vi "HFRR ADV v07.vi"() -> ()   [LabVIEW 2025] (continued)
        n800 = local write "CAMERA ROI MIN TEMP"(TRUE ("CAMERA ROI MIN TEMP")) -> ()
      }
      frame "Compare Files" {
        n801 = local read "LIVE FEED MIN TEMP"() -> (w1178:bool)
        n802 = local write "LIVE FEED MAX TEMP"(TRUE ("LIVE FEED MAX TEMP")) -> ()
        n803 = local read "CAMERA ROI MIN TEMP"() -> (w1176:bool)
        n804 = case shown="True" w1178 {
          selector: w1178 -> [_ w1185]
          frame False {
          }
          frame True {
            n805 = Not(x=w1185) -> (.not. x?=w1184:bool)
            n806 = local write "LIVE FEED MIN TEMP"(w1184) -> ()
            n807 = call "CAMERA LIVE FEED FGV.vi"("Enum - Menu"=CAMERA_LIVE_FEED_ENUM."CAMERA MINIMIZE") -> ()  [unwired: 9 in, 2 out]
          }
        }
        n808 = case shown="True" w1176 {
          selector: w1176 -> [_ w1182]
          frame False {
          }
          frame True {
            n809 = Not(x=w1182) -> (.not. x?=w1181:bool)
            n810 = local write "CAMERA ROI MIN TEMP"(w1181) -> ()
            n811 = call "IMAGE ANALYSIS.vi"("Enum"=POST_ANALYSIS_ENUM."MINIMIZE UI") -> ()  [unwired: 9 in, 2 out]
          }
        }
        n812 = local write "CAMERA ROI MAX TEMP"(TRUE ("CAMERA ROI MAX TEMP")) -> ()
      }
      frame "About" {
        n813 = local read "LIVE FEED MIN TEMP"() -> (w1188:bool)
        n814 = local write "LIVE FEED MAX TEMP"(TRUE ("LIVE FEED MAX TEMP")) -> ()
        n815 = local read "CAMERA ROI MIN TEMP"() -> (w1187:bool)
        n816 = case shown="True" w1188 {
          selector: w1188 -> [_ w1195]
          frame False {
          }
          frame True {
            n817 = Not(x=w1195) -> (.not. x?=w1194:bool)
            n818 = local write "LIVE FEED MIN TEMP"(w1194) -> ()
            n819 = call "CAMERA LIVE FEED FGV.vi"("Enum - Menu"=CAMERA_LIVE_FEED_ENUM."CAMERA MINIMIZE") -> ()  [unwired: 9 in, 2 out]
          }
        }
        n820 = case shown="True" w1187 {
          selector: w1187 -> [_ w1192]
          frame False {
          }
          frame True {
            n821 = Not(x=w1192) -> (.not. x?=w1191:bool)
            n822 = local write "CAMERA ROI MIN TEMP"(w1191) -> ()
            n823 = call "IMAGE ANALYSIS.vi"("Enum"=POST_ANALYSIS_ENUM."MINIMIZE UI") -> ()  [unwired: 9 in, 2 out]
          }
        }
        n824 = local write "CAMERA ROI MAX TEMP"(TRUE ("CAMERA ROI MIN TEMP")) -> ()
      }
      frame "Advance" {
        n825 = local read "LIVE FEED MIN TEMP"() -> (w1198:bool)
        n826 = local write "LIVE FEED MAX TEMP"(TRUE ("LIVE FEED MAX TEMP")) -> ()
        n827 = local read "CAMERA ROI MIN TEMP"() -> (w1196:bool)
        n828 = case shown="True" w1198 {
          selector: w1198 -> [_ w1205]
          frame False {
          }
          frame True {
            n829 = Not(x=w1205) -> (.not. x?=w1204:bool)
            n830 = local write "LIVE FEED MIN TEMP"(w1204) -> ()
            n831 = call "CAMERA LIVE FEED FGV.vi"("Enum - Menu"=CAMERA_LIVE_FEED_ENUM."CAMERA MINIMIZE") -> ()  [unwired: 9 in, 2 out]
          }
        }
        n832 = local write "CAMERA ROI MAX TEMP"(TRUE ("CAMERA ROI MAX TEMP")) -> ()
        n833 = case shown="True" w1196 {
          selector: w1196 -> [_ w1202]
          frame False {
          }
          frame True {
            n834 = Not(x=w1202) -> (.not. x?=w1201:bool)
            n835 = local write "CAMERA ROI MIN TEMP"(w1201) -> ()
            n836 = call "IMAGE ANALYSIS.vi"("Enum"=POST_ANALYSIS_ENUM."MINIMIZE UI") -> ()  [unwired: 9 in, 2 out]
          }
        }
      }
      frame "Mooha" {
        n837 = local read "LIVE FEED MIN TEMP"() -> (w1208:bool)
        n838 = local write "LIVE FEED MAX TEMP"(TRUE ("LIVE FEED MAX TEMP")) -> ()
        n839 = local read "CAMERA ROI MIN TEMP"() -> (w1206:bool)
        n840 = case shown="True" w1208 {
          selector: w1208 -> [_ w1215]
          frame False {
          }
          frame True {
            n841 = Not(x=w1215) -> (.not. x?=w1214:bool)
            n842 = local write "LIVE FEED MIN TEMP"(w1214) -> ()
            n843 = call "CAMERA LIVE FEED FGV.vi"("Enum - Menu"=CAMERA_LIVE_FEED_ENUM."CAMERA MINIMIZE") -> ()  [unwired: 9 in, 2 out]
          }
        }
        n844 = local write "CAMERA ROI MAX TEMP"(TRUE ("CAMERA ROI MAX TEMP")) -> ()
        n845 = case shown="True" w1206 {
          selector: w1206 -> [_ w1212]
          frame False {
          }
          frame True {
            n846 = Not(x=w1212) -> (.not. x?=w1211:bool)
            n847 = local write "CAMERA ROI MIN TEMP"(w1211) -> ()
            n848 = call "IMAGE ANALYSIS.vi"("Enum"=POST_ANALYSIS_ENUM."MINIMIZE UI") -> ()  [unwired: 9 in, 2 out]
          }
        }
      }
    }
    n849 = local read "Auto Start Test"() -> (w958:bool)
    n850 = case shown="True" "sign in temp" {
      frame False {
      }
      frame True {
        w994 = 1 ("y")
        n851 = local read "USERNAME"() -> (w1000:string)
        n852 = local read "USER ID"() -> (w997:string)
        n853 = call <vilib>:"Trim Whitespace.vi"("string"=w997) -> ("trimmed string"=w998:string)  [unwired: 1 in]
        n854 = call <vilib>:"Trim Whitespace.vi"("string"=w1000) -> ("trimmed string"=w999:string)  [unwired: 1 in]
        n855 = String Length(string=w998) -> (length=w995:i32)
        n856 = String Length(string=w999) -> (length=w996:i32)
        n857 = Greater?(x=w995, y=w994) -> (0:w992:bool)
        n858 = Greater?(x=w996, y=w994) -> (0:w993:bool)
        n859 = And(x=w993, y=w992) -> (x .and. y?=w991:bool)
        n860 = case shown="True" w991 {
          frame False {
            n861 = property on="Sign In" class="Bool (strict)"("DisabledEnum"=T15."Disabled" ("Disabled")) -> ()  [unwired: 2 in, 2 out]
          }
          frame True {
            n862 = property on="Sign In" class="Bool (strict)"("DisabledEnum"=T15."Enabled" ("Disabled")) -> ()  [unwired: 2 in, 2 out]
          }
        }
      }
    }
    n863 = local read "Air Temperature"() -> (w975:bool)
    n864 = local read "Coefficient Of Friction"() -> (w976:bool)
    n865 = case shown="False" w958 {
      frame False {
        n866 = local read "Auto stop temp"() -> (w988:bool)
        n867 = case shown="True" w988 {
          frame False {
          }
          frame True {
            n868 = local write "Auto Start Temp"(FALSE ("Auto Start Temp")) -> ()
          }
        }
      }
      frame True {
        "Auto stop temp" <- TRUE ("Auto stop temp")
      }
    }
    n869 = local read "Humidity"() -> (w974:bool)
    n870 = case shown="\"Numeric Display\", Default" "Num/Graph" {
      frame "Numeric Display", Default {
        n871 = property on="Single - Graph" class="Ring (strict)"("Visible"=FALSE) -> ()  [unwired: 2 in, 2 out]
        n872 = property on="Single/Multiple" class="RadioBtnsControl (strict)"("Visible"=FALSE) -> ()  [unwired: 2 in, 2 out]
        n873 = local write "Main Tab Display"(T4."Dashboard 1" ("Main Tab Display")) -> ()
      }
      frame "Graph Display" {
        n874 = property on="Single/Multiple" class="RadioBtnsControl (strict)"("Visible"=TRUE) -> ()  [unwired: 2 in, 2 out]
        n875 = case shown="\"Multiple\"" "Single/Multiple" {
          frame "Single ", Default {
            n876 = property on="Single - Graph" class="Ring (strict)"("Visible"=TRUE) -> ()  [unwired: 2 in, 2 out]
            n877 = local write "Main Tab Display"(T4."Dashboard 3" ("Main Tab Display")) -> ()
          }
          frame "Multiple" {
            n878 = property on="Single - Graph" class="Ring (strict)"("Visible"=FALSE) -> ()  [unwired: 2 in, 2 out]
            n879 = local write "Main Tab Display"(T4."Dashboard 2" ("Main Tab Display")) -> ()
          }
        }
      }
    }
    n880 = case shown="True" w984 {
      selector: w984 -> [_ w1321]
      frame False {
      }
      frame True {
        n881 = Not(x=w1321) -> (.not. x?=w1320:bool)
        n882 = local write "Sign In"(w1320) -> ()
        n883 = local write "Main Dashboard Buttons"(T1."Test Setup" ("Main Dashboard Buttons")) -> ()
      }
    }
    n884 = case shown="\"HOME\"" w985 {
      frame "HOME" {
        n885 = local write "main tab sub"(enum32{"Page 1", "Page 2"}."Page 1" ("main tab sub")) -> ()
      }
      frame Default {
        n886 = local write "main tab sub"(enum32{"Page 1", "Page 2"}."Page 2" ("main tab sub")) -> ()
      }
    }
    n887 = local read "Stroke"() -> (w973:bool)
    n888 = local read "USERNAME"() -> (w979:string)
    n889 = local read "USER ID"() -> (w978:string)
    n890 = case shown="True" w976 {
      selector: w976 -> [_ w1255]
      frame False {
      }
      frame True {
        n891 = Not(x=w1255) -> (.not. x?=w1254:bool)
        n892 = local write "Coefficient Of Friction"(w1254) -> ()
        n893 = local write "Tab Control 2"(T6."Coefficient Of Friction" ("Tab Control 2")) -> ()
      }
    }
    n894 = case shown="True" w975 {
      selector: w975 -> [_ w1252]
      frame False {
      }
      frame True {
        n895 = Not(x=w1252) -> (.not. x?=w1250:bool)
        n896 = local write "Air Temperature"(w1250) -> ()
        n897 = local write "Tab Control 2"(T6."Air Temperature" ("Tab Control 2")) -> ()
      }
    }
    n898 = local write "Operator ID"(w978) -> ()
    n899 = case shown="True" w973 {
      selector: w973 -> [_ w1246]
      frame False {
      }
      frame True {
        n900 = Not(x=w1246) -> (.not. x?=w1244:bool)
        n901 = local write "Stroke"(w1244) -> ()
        n902 = local write "Tab Control 2"(T6."Stroke" ("Tab Control 2")) -> ()
      }
    }
    n903 = local write "tested by"(w979) -> ()
    n904 = case shown="True" w974 {
      selector: w974 -> [_ w1249]
      frame False {
      }
      frame True {
        n905 = Not(x=w1249) -> (.not. x?=w1247:bool)
        n906 = local write "Humidity"(w1247) -> ()
        n907 = local write "Tab Control 2"(T6."Humidity" ("Tab Control 2")) -> ()
      }
    }
    n908 = case shown="\"Calibration\"" "Main Dashboard Buttons" {
      tunnel: [T2."HOME" ("Main Tab") T2."Test Setup" ("Main Tab") T2."Calibration" ("Main Tab") T2."Acquire" ("Main Tab") T2."Adv Scar" ("Main Tab") T2."Adv Scar Report" ("Main Tab") T2."Compare Files" ("Main Tab") T2."About" ("Main Tab") T2."Advance" ("Main Tab")] -> w957
      frame "Home", Default {
      }
      frame "Test Setup" {
      }
      frame "Calibration" {
      }
      frame "Dashboard" {
      }
      frame "Imaging" {
      }
      frame "Report" {
      }
      frame "Analysis" {
      }
      frame "About" {
      }
      frame "Advance" {
      }
    }
    n909 = Wait (ms)(milliseconds to wait=u32 100) -> ()  [unwired: 1 out]
    n910 = local read "Main Tab Display"() -> (w977:T4)
    n911 = local write "Main Tab"(w957) -> ()
    n912 = case shown="\"Dashboard 3\"" w977 {
      frame "Dashboard 1", Default {
        n913 = property on="Reset Graph" class="Bool (strict)"("Visible"=FALSE) -> ()  [unwired: 2 in, 2 out]
      }
      frame "Dashboard 2" {
        n914 = property on="Reset Graph" class="Bool (strict)"("Visible"=TRUE) -> ()  [unwired: 2 in, 2 out]
      }
      frame "Dashboard 3" {
        n915 = property on="Reset Graph" class="Bool (strict)"("Visible"=TRUE) -> ()  [unwired: 2 in, 2 out]
      }
    }
    n916 = local read "SCAR MEASURMENT"() -> (w965:enum32{"Auto Scar", "Manual Scar"})
    n917 = local read "Humidity"() -> (w980:bool)
    n918 = local read "Cap Live Image"() -> (w962:bool)
    n919 = local read "Sample Temperature"() -> (w972:bool)
    n920 = local read "Air Temp vs Humidity"() -> (w970:bool)
    n921 = local read "Frequency"() -> (w971:bool)
    n922 = case shown="False" w980 {
      frame False {
        n923 = local write "Humidity On Command"(TRUE ("Humidity On Command")) -> ()
        n924 = case shown="True" "Humidity Off Command" {
          selector: "Humidity Off Command" -> [_ w1262]
          frame False {
          }
          frame True {
            n925 = stacked-sequence {
              frame #0 {
                n926 = local read "WriteHumidity"() -> (w1264:string[])
                n927 = Insert Into Array(array=w1264, new element="R;1" ("new element/subarray")) -> (w1265:string[])  [unwired: 1 in]
                n928 = local write "WriteHumidity"(w1265) -> ()
              }
              frame #1 {
                n929 = Wait (ms)(milliseconds to wait=u32 2000) -> ()  [unwired: 1 out]
              }
              frame #2 {
                n930 = local read "EVENT LOG"() -> (w1271:string)
                n931 = local read "WriteHumidity"() -> (w1268:string[])
                n932 = call "Event Log.vi"("Content"="Humidity Control Off" ("string"), "EVENT LOG"=w1271) -> ("EVENT LOG"=w1272:string)  [unwired: 8 in, 1 out]
                n933 = local write "EVENT LOG"(w1272) -> ()
                n934 = Insert Into Array(array=w1268, new element="R;1" ("new element/subarray")) -> (w1269:string[])  [unwired: 1 in]
                n935 = local write "WriteHumidity"(w1269) -> ()
              }
            }
            n936 = Not(x=w1262) -> (.not. x?=w1261:bool)
            n937 = local write "Humidity Off Command"(w1261) -> ()
          }
        }
      }
      frame True {
        n938 = local write "Humidity Off Command"(TRUE ("Humidity Off Command")) -> ()
        n939 = case shown="False" "Humidity On Command" {
          selector: "Humidity On Command" -> [_ w1276]
          frame False {
          }
          frame True {
            n940 = stacked-sequence {
              frame #0 {
                n941 = local read "Set Rh"() -> (w1282:dbl)
                n942 = Number To Fractional String(number=w1282, precision (6)=i16 2) -> (F-format string=w1283:string)  [unwired: 2 in]
                n943 = local read "WriteHumidity"() -> (w1280:string[])
                n944 = Concatenate Strings("M;" ("new element/subarray"), w1283) -> (w1281:string)
                n945 = Insert Into Array(array=w1280, new element=w1281) -> (w1279:string[])  [unwired: 1 in]
                n946 = local write "WriteHumidity"(w1279) -> ()
              }
              frame #1 {
                n947 = Wait (ms)(milliseconds to wait=u32 1500) -> ()  [unwired: 1 out]
              }
              frame #2 {
                (unwired) "% RH" ("string")
                (unwired) i16 2 ("precision (6)")
                (unwired) "M;" ("new element/subarray")
                n948 = local read "Set Rh"() -> (w1290:dbl)
                n949 = Number To Fractional String(number=w1290, precision (6)=i16 2) -> (F-format string=w1287:string)  [unwired: 2 in]
                n950 = local read "WriteHumidity"() -> (w1292:string[])
                n951 = Concatenate Strings("M;" ("new element/subarray"), w1287) -> (w1291:string)
                n952 = Concatenate Strings("Humidity Set to : " ("string"), w1287, "% RH" ("string")) -> (w1285:string)
                n953 = Insert Into Array(array=w1292, new element=w1291) -> (w1293:string[])  [unwired: 1 in]
                n954 = disable-structure shown="Enabled" {
                  frame Enabled {
                    n955 = local read "EVENT LOG"() -> (w1296:string)
                    n956 = call "Event Log.vi"("Content"="Humidity Control On", "EVENT LOG"=w1296) -> ("EVENT LOG"=w1297:string)  [unwired: 8 in, 1 out]
                    n957 = local write "EVENT LOG"(w1297) -> ()
                  }
                  frame Disabled {
                  }
                }
                n958 = disable-structure shown="Enabled" {
                  disable-tunnel: w1285 -> [_ _]
                  frame Enabled {
                    n959 = local read "EVENT LOG"() -> (w1299:string)
                    n960 = call "Event Log.vi"("Content"="Humidity Control On", "EVENT LOG"=w1299) -> ("EVENT LOG"=w1300:string)  [unwired: 8 in, 1 out]
                    n961 = local write "EVENT LOG"(w1300) -> ()
                  }
                  frame Disabled {
                  }
                }
                n962 = local write "WriteHumidity"(w1293) -> ()
              }
            }
            n963 = Not(x=w1276) -> (.not. x?=w1275:bool)
            n964 = local write "Humidity On Command"(w1275) -> ()
          }
        }
      }
    }
    n965 = Equal?(x=w965, y=enum32{"Auto Scar", "Manual Scar"}."Auto Scar" ("SCAR MEASURMENT")) -> (x = y?=w961:bool)
    n966 = And(x=w962, y=w961) -> (x .and. y?=w963:bool)
    n967 = local read "TEST STANDARD"() -> (w968:T3)
    n968 = case shown="True" w963 {
      selector: w963 -> [_ w1061]
      tunnel: errorcluster {"status"=FALSE, "code"=0, "source"=""} ("error in (no error) 3") -> [_ w1062]
      frame False {
      }
      frame True {
        n969 = stacked-sequence {
          tunnel: w1062 -> [_ _ _ _ _ _ _ w1110]
          tunnel: w1061 -> [_ _ _ _ _ w1091 _ _]
          frame #0 {
            n970 = call "CAMERA LIVE FEED FGV.vi"("Enum - Menu"=CAMERA_LIVE_FEED_ENUM."CAMERA MINIMIZE") -> ()  [unwired: 9 in, 2 out]
          }
          frame #1 {
            n971 = property on="Auto Scar Check  2" class="Clust (strict)"("Visible"=TRUE) -> ()  [unwired: 2 in, 2 out]
          }
          frame #2 {
            n972 = String To Path(string="C:\\LAB-IQ\\Image Calibrate v01.dcf") -> (path=w1067:path)
            n973 = Open/Create/Replace File ("Open File")(file path (use dialog)=w1067) -> (refnum out=w1068:refnum<file>)  [unwired: 5 in, 2 out]
            n974 = for {
              N: 4 -> [_]
              tunnel: w1068 -> [w1074]
              i -> [w1070]
              n975 = Read from Text File ("Read File")(file (use dialog)=w1074) -> (text=w1075:string)  [unwired: 3 in, 3 out]
              n976 = String Subset(string=w1075, offset (0)=6, length (rest)=10 ("length (rest)")) -> (substring=w1071:string)
              n977 = Fract/Exp String To Number(string=w1071) -> (number=w1069:dbl)  [unwired: 3 in, 1 out]
              n978 = case shown="0" w1070 {
                tunnel: w1069 -> [w1076 w1077 _ w1078 _]
                frame 0 {
                  "5x Gain" <- w1076
                }
                frame 1 {
                  "10x Gain" <- w1077
                }
                frame 2 {
                }
                frame 3 {
                  "100x gain" <- w1078
                }
                frame 4, Default {
                }
              }
            }
          }
          frame #3 {
            n979 = local read "FILE 3"() -> (w1084:string)
            n980 = call <vilib>:"Trim Whitespace.vi"("string"="C:\\LAB-IQ\\images\\") -> ("trimmed string"=w1086:string)  [unwired: 1 in]
            n981 = String To Path(string=w1086) -> (path=w1085:path)
            n982 = Concatenate Strings(w1084, ".png" ("string")) -> (w1083:string)
            n983 = Build Path(base path=w1085, name or relative path=w1083) -> (appended path=w1081:path)
            "Image path" <- w1081
            n984 = Path To String(path=w1081) -> (string=w1080:string)
            n985 = call "CAMERA LIVE FEED FGV.vi"("Enum - Menu"=CAMERA_LIVE_FEED_ENUM."CAMERA SAVE", "Image Path"=w1080) -> ()  [unwired: 8 in, 2 out]
          }
          frame #4 {
            n986 = One Button Dialog(message="Image saved successfully") -> ()  [unwired: 1 in, 1 out]
          }
          frame #5 {
            n987 = local read "TEST STANDARD"() -> (w1090:T3)
            n988 = local read "Magnification len live scar"() -> (w1102:string)
            n989 = Not(x=w1091) -> (.not. x?=w1092:bool)
            n990 = local write "Cap Live Image"(w1092) -> ()
            n991 = case shown="\"ISO 12156\"" w1090 {
              tunnel: ["ASTM D6079" "ISO 12156"] -> w1089
              frame "ASTM D6079", Default {
              }
              frame "ISO 12156" {
              }
            }
            n992 = case shown="\"5x\", Default" w1102 {
              tunnel: [w1105 w1106] -> w1101
              frame "5x", Default {
                n993 = local read "5x Gain"() -> (w1105:dbl)
              }
              frame "10x" {
                # "5x"
                n994 = local read "10x Gain"() -> (w1106:dbl)
              }
            }
            n995 = local read "Image path"() -> (w1100:path)
            n996 = local read "FILE 3"() -> (w1093:string)
            n997 = call "EDGE DETCTION.vi"("GAIN VALUE"=w1101, "Image Path"=w1100) -> ("error out"=w1099:errorcluster, "return value"=w1098:cluster{string, string, dbl, dbl, dbl})  [unwired: 8 in]
            n998 = Bundle By Name(cluster=T21 {"File Name"="", "Test Method"="", "Operator"="", "Fuel Description"="", "Date and time"=""} ("Main Ref"), "File Name"=w1093, "Test Method"=w1089) -> (w1094:T21)
            n999 = call "duf file read.vi"("error in (no error)"=w1099, "Main Ref"=w1094) -> ("error out"=w1097:errorcluster, "Main Ref 2"=w1095:T21)  [unwired: 8 in]
            n1000 = call "EDGE DETECTION REPORT.vi"("error in (no error)"=w1097, "return value 2"=w1098, "Main Ref"=w1095) -> ()  [unwired: 8 in, 1 out]
          }
          frame #6 {
            n1001 = property on="Auto Scar Check  2" class="Clust (strict)"("Visible"=FALSE) -> ()  [unwired: 2 in, 2 out]
          }
          frame #7 {
            n1002 = call "CAMERA LIVE FEED FGV.vi"("Enum - Menu"=CAMERA_LIVE_FEED_ENUM."CAMERA MINIMIZE", "error in (no error)"=w1110) -> ()  [unwired: 8 in, 2 out]
            n1003 = local write "Main Dashboard Buttons"(T1."Home" ("Main Dashboard Buttons")) -> ()
            n1004 = local write "Main Tab"(T2."HOME" ("Main Tab")) -> ()
          }
        }
      }
    }
    n1005 = local read "Heater Button"() -> (w969:bool)
    n1006 = case shown="True" w970 {
      selector: w970 -> [_ w1237]
      frame False {
      }
      frame True {
        n1007 = Not(x=w1237) -> (.not. x?=w1235:bool)
        n1008 = local write "Air Temp vs Humidity"(w1235) -> ()
        n1009 = local write "Tab Control 2"(T6."Air Temp vs Rh" ("Tab Control 2")) -> ()
      }
    }
    n1010 = case shown="True" w971 {
      selector: w971 -> [_ w1240]
      frame False {
      }
      frame True {
        n1011 = Not(x=w1240) -> (.not. x?=w1238:bool)
        n1012 = local write "Frequency"(w1238) -> ()
        n1013 = local write "Tab Control 2"(T6."Frequency" ("Tab Control 2")) -> ()
      }
    }
    n1014 = case shown="True" w972 {
      selector: w972 -> [_ w1243]
      frame False {
      }
      frame True {
        n1015 = Not(x=w1243) -> (.not. x?=w1241:bool)
        n1016 = local write "Sample Temperature"(w1241) -> ()
        n1017 = local write "Tab Control 2"(T6."Sample Temperature" ("Tab Control 2")) -> ()
      }
    }
    n1018 = case shown="\"Custom\"" w968 {
      frame "ASTM D6079", Default {
        w1216 = "ASTM D6079 TEST CONDITIONS" ("Standard 2")
        n1019 = local write "Standard 2"(w1216) -> ()
        n1020 = local write "Standard"(w1216) -> ()
      }
      frame "ISO 12156" {
        w1217 = "ISO 12156 TEST CONDITIONS" ("Standard 2")
        n1021 = local write "Standard 2"(w1217) -> ()
        n1022 = local write "Standard"(w1217) -> ()
      }
      frame "CEC F-096-A-06" {
        w1218 = "CEC F-096-A-06 TEST CONDITIONS" ("Standard 2")
        n1023 = local write "Standard 2"(w1218) -> ()
        n1024 = local write "Standard"(w1218) -> ()
      }
      frame "Custom" {
        w1219 = "CUSTOM TEST CONDITIONS" ("Standard 2")
        n1025 = local write "Standard 2"(w1219) -> ()
        n1026 = local write "Standard"(w1219) -> ()
      }
    }
    n1027 = case shown="False" w969 {
      frame False {
        n1028 = local write "Temperature On Command"(TRUE ("Temperature On Command")) -> ()
        n1029 = case shown="True" "Temperature Off Command" {
          selector: "Temperature Off Command" -> [_ w1223]
          frame False {
          }
          frame True {
            n1030 = Not(x=w1223) -> (.not. x?=w1222:bool)
            n1031 = local read "EVENT LOG"() -> (w1226:string)
            n1032 = local write "Temperature Off Command"(w1222) -> ()
            n1033 = call "Event Log.vi"("Content"="Heater Off", "EVENT LOG"=w1226) -> ("EVENT LOG"=w1225:string)  [unwired: 8 in, 1 out]
            n1034 = local write "EVENT LOG"(w1225) -> ()
          }
        }
      }
      frame True {
        n1035 = local write "Temperature Off Command"(TRUE ("Temperature Off Command")) -> ()
        n1036 = case shown="True" "Temperature On Command" {
          selector: "Temperature On Command" -> [_ w1230]
          frame False {
          }
          frame True {
            n1037 = Not(x=w1230) -> (.not. x?=w1229:bool)
            n1038 = local write "Temperature On Command"(w1229) -> ()
            n1039 = disable-structure shown="Enabled" {
              disable-tunnel: "Heater On" -> [w1232 _]
              frame Enabled {
                n1040 = local read "EVENT LOG"() -> (w1233:string)
                n1041 = call "Event Log.vi"("Content"=w1232, "EVENT LOG"=w1233) -> ("EVENT LOG"=w1234:string)  [unwired: 8 in, 1 out]
                n1042 = local write "EVENT LOG"(w1234) -> ()
              }
              frame Disabled {
              }
            }
          }
        }
      }
    }
    n1043 = local read "Main Tab"() -> (w960:T2)
    n1044 = case shown="\"About\"" w960 {
      frame "HOME", Default {
        w1005 = T15."Enabled" ("Disabled")
        n1045 = local read "Service Password enable"() -> (w1004:bool)
        n1046 = property on="Analysis" class="Bool (strict)"("DisabledEnum"=w1005) -> ()  [unwired: 2 in, 2 out]
        n1047 = property on="Report" class="Bool (strict)"("DisabledEnum"=w1005) -> ()  [unwired: 2 in, 2 out]
        n1048 = property on="Imaging" class="Bool (strict)"("DisabledEnum"=w1005) -> ()  [unwired: 2 in, 2 out]
        n1049 = property on="Dashboard" class="Bool (strict)"("DisabledEnum"=w1005) -> ()  [unwired: 2 in, 2 out]
        n1050 = property on="Test Setup" class="Bool (strict)"("DisabledEnum"=w1005) -> ()  [unwired: 2 in, 2 out]
        n1051 = property on="Home" class="Bool (strict)"("DisabledEnum"=w1005) -> ()  [unwired: 2 in, 2 out]
        n1052 = property on="Main Dashboard Buttons" class="RadioBtnsControl (strict)"("DisabledEnum"=w1005) -> ()  [unwired: 2 in, 2 out]
        n1053 = case shown="True" w1004 {
          tunnel: [T15."Disabled" ("Disabled") T15."Enabled" ("Disabled")] -> w1003
          frame False {
          }
          frame True {
          }
        }
        n1054 = property on="About" class="Bool (strict)"("DisabledEnum"=w1003) -> ()  [unwired: 2 in, 2 out]
      }
      frame "Test Setup" {
        w1010 = T15."Enabled" ("Disabled")
        n1055 = local read "Service Password enable"() -> (w1009:bool)
        n1056 = property on="Report" class="Bool (strict)"("DisabledEnum"=w1010) -> ()  [unwired: 2 in, 2 out]
        n1057 = property on="Home" class="Bool (strict)"("DisabledEnum"=w1010) -> ()  [unwired: 2 in, 2 out]
        n1058 = property on="Analysis" class="Bool (strict)"("DisabledEnum"=w1010) -> ()  [unwired: 2 in, 2 out]
        n1059 = property on="Imaging" class="Bool (strict)"("DisabledEnum"=w1010) -> ()  [unwired: 2 in, 2 out]
        n1060 = property on="Dashboard" class="Bool (strict)"("DisabledEnum"=T15."Disabled" ("Disabled")) -> ()  [unwired: 2 in, 2 out]
        n1061 = property on="Test Setup" class="Bool (strict)"("DisabledEnum"=w1010) -> ()  [unwired: 2 in, 2 out]
        n1062 = case shown="True" w1009 {
          tunnel: [T15."Disabled" ("Disabled") T15."Enabled" ("Disabled")] -> w1008
          frame False {
          }
          frame True {
          }
        }
        n1063 = property on="About" class="Bool (strict)"("DisabledEnum"=w1008) -> ()  [unwired: 2 in, 2 out]
      }
      frame "Adv Scar" {
        w1017 = T15."Enabled" ("Disabled")
        n1064 = property on="Report" class="Bool (strict)"("DisabledEnum"=w1017) -> ()  [unwired: 2 in, 2 out]
        n1065 = property on="Home" class="Bool (strict)"("DisabledEnum"=w1017) -> ()  [unwired: 2 in, 2 out]
        n1066 = property on="Analysis" class="Bool (strict)"("DisabledEnum"=w1017) -> ()  [unwired: 2 in, 2 out]
        n1067 = property on="Imaging" class="Bool (strict)"("DisabledEnum"=w1017) -> ()  [unwired: 2 in, 2 out]
        n1068 = property on="Dashboard" class="Bool (strict)"("DisabledEnum"=T15."Disabled" ("Disabled")) -> ()  [unwired: 2 in, 2 out]
        n1069 = property on="Test Setup" class="Bool (strict)"("DisabledEnum"=w1017) -> ()  [unwired: 2 in, 2 out]
        n1070 = local read "Service Password enable"() -> (w1015:bool)
        n1071 = case shown="True" w1015 {
          tunnel: [T15."Disabled" ("Disabled") T15."Enabled" ("Disabled")] -> w1014
          frame False {
          }
          frame True {
          }
        }
        n1072 = property on="About" class="Bool (strict)"("DisabledEnum"=w1014) -> ()  [unwired: 2 in, 2 out]
      }
      frame "Adv Scar Report" {
        w1022 = T15."Enabled" ("Disabled")
        n1073 = property on="Report" class="Bool (strict)"("DisabledEnum"=w1022) -> ()  [unwired: 2 in, 2 out]
        n1074 = property on="Home" class="Bool (strict)"("DisabledEnum"=w1022) -> ()  [unwired: 2 in, 2 out]
        n1075 = property on="Analysis" class="Bool (strict)"("DisabledEnum"=w1022) -> ()  [unwired: 2 in, 2 out]
        n1076 = property on="Imaging" class="Bool (strict)"("DisabledEnum"=w1022) -> ()  [unwired: 2 in, 2 out]
        n1077 = property on="Dashboard" class="Bool (strict)"("DisabledEnum"=T15."Disabled" ("Disabled")) -> ()  [unwired: 2 in, 2 out]
        n1078 = property on="Test Setup" class="Bool (strict)"("DisabledEnum"=w1022) -> ()  [unwired: 2 in, 2 out]
        n1079 = local read "Service Password enable"() -> (w1021:bool)
        n1080 = case shown="True" w1021 {
          tunnel: [T15."Disabled" ("Disabled") T15."Enabled" ("Disabled")] -> w1020
          frame False {
          }
          frame True {
          }
        }
        n1081 = property on="About" class="Bool (strict)"("DisabledEnum"=w1020) -> ()  [unwired: 2 in, 2 out]
      }
      frame "Compare Files" {
        w1028 = T15."Enabled" ("Disabled")
        n1082 = local read "Service Password enable"() -> (w1027:bool)
        n1083 = property on="Report" class="Bool (strict)"("DisabledEnum"=w1028) -> ()  [unwired: 2 in, 2 out]
        n1084 = property on="Home" class="Bool (strict)"("DisabledEnum"=w1028) -> ()  [unwired: 2 in, 2 out]
        n1085 = property on="Analysis" class="Bool (strict)"("DisabledEnum"=w1028) -> ()  [unwired: 2 in, 2 out]
        n1086 = property on="Imaging" class="Bool (strict)"("DisabledEnum"=w1028) -> ()  [unwired: 2 in, 2 out]
        n1087 = property on="Dashboard" class="Bool (strict)"("DisabledEnum"=T15."Disabled" ("Disabled")) -> ()  [unwired: 2 in, 2 out]
        n1088 = property on="Test Setup" class="Bool (strict)"("DisabledEnum"=w1028) -> ()  [unwired: 2 in, 2 out]
        n1089 = case shown="True" w1027 {
          tunnel: [T15."Disabled" ("Disabled") T15."Enabled" ("Disabled")] -> w1026
          frame False {
          }
          frame True {
          }
        }
        n1090 = property on="About" class="Bool (strict)"("DisabledEnum"=w1026) -> ()  [unwired: 2 in, 2 out]
      }
      frame "Acquire" {
        n1091 = local read "Service Password enable"() -> (w1032:bool)
        n1092 = local read "Auto Start Test"() -> (w1034:bool)
        n1093 = property on="Test Setup" class="Bool (strict)"("DisabledEnum"=T15."Disabled" ("Disabled")) -> ()  [unwired: 2 in, 2 out]
        n1094 = local read "RUN"() -> (w1036:bool)
        n1095 = case shown="True" w1032 {
          tunnel: [T15."Disabled" ("Disabled") T15."Enabled" ("Disabled")] -> w1033
          frame False {
          }
          frame True {
          }
        }
        n1096 = Or(x=w1036, y=w1034) -> (x .or. y?=w1035:bool)
        n1097 = case shown="True" w1035 {
          tunnel: [T15."Enabled" ("Disabled") T15."Disabled" ("Disabled")] -> w1038
          frame False {
          }
          frame True {
          }
        }
        n1098 = property on="About" class="Bool (strict)"("DisabledEnum"=w1033) -> ()  [unwired: 2 in, 2 out]
        n1099 = property on="Report" class="Bool (strict)"("DisabledEnum"=w1038) -> ()  [unwired: 2 in, 2 out]
        n1100 = property on="Home" class="Bool (strict)"("DisabledEnum"=w1038) -> ()  [unwired: 2 in, 2 out]
        n1101 = property on="Analysis" class="Bool (strict)"("DisabledEnum"=w1038) -> ()  [unwired: 2 in, 2 out]
        n1102 = property on="Imaging" class="Bool (strict)"("DisabledEnum"=w1038) -> ()  [unwired: 2 in, 2 out]
        n1103 = property on="Dashboard" class="Bool (strict)"("DisabledEnum"=w1038) -> ()  [unwired: 2 in, 2 out]
      }
      frame "About" {
        n1104 = local read "FILE"() -> (w1051:string)
        n1105 = local read "TEST FILE NAM,E SAVED"() -> (w1044:bool)
        n1106 = call <vilib>:"Trim Whitespace.vi"("string"=w1051) -> ("trimmed string"=w1050:string)  [unwired: 1 in]
        n1107 = local read "Auto Start Test"() -> (w1054:bool)
        n1108 = String Length(string=w1050) -> (length=w1049:i32)
        n1109 = Greater?(x=w1049, y=1) -> (0:w1046:bool)
        n1110 = And(x=w1046, y=w1044) -> (x .and. y?=w1045:bool)
        n1111 = local read "RUN"() -> (w1056:bool)
        n1112 = case shown="True" w1045 {
          tunnel: [T15."Disabled" ("Disabled") T15."Enabled" ("Disabled")] -> w1047
          frame False {
          }
          frame True {
          }
        }
        n1113 = Or(x=w1056, y=w1054) -> (x .or. y?=w1055:bool)
        n1114 = property on="About" class="Bool (strict)"("DisabledEnum"=T15."Enabled" ("Disabled")) -> ()  [unwired: 2 in, 2 out]
        n1115 = case shown="False" w1055 {
          tunnel: [T15."Enabled" ("Disabled") T15."Disabled" ("Disabled")] -> w1053
          frame False {
          }
          frame True {
          }
        }
        n1116 = property on="Dashboard" class="Bool (strict)"("DisabledEnum"=w1047) -> ()  [unwired: 2 in, 2 out]
        n1117 = property on="Test Setup" class="Bool (strict)"("DisabledEnum"=T15."Disabled" ("Disabled")) -> ()  [unwired: 2 in, 2 out]
        n1118 = property on="Report" class="Bool (strict)"("DisabledEnum"=w1053) -> ()  [unwired: 2 in, 2 out]
        n1119 = property on="Home" class="Bool (strict)"("DisabledEnum"=w1053) -> ()  [unwired: 2 in, 2 out]
        n1120 = property on="Analysis" class="Bool (strict)"("DisabledEnum"=w1053) -> ()  [unwired: 2 in, 2 out]
        n1121 = property on="Imaging" class="Bool (strict)"("DisabledEnum"=w1053) -> ()  [unwired: 2 in, 2 out]
      }
    }
    n1122 = local read "Quit"() -> (w987:bool)
    "Single" <- "Single - Graph"
  }
  n1123 = disable-structure shown="Disabled" {
    disable-tunnel: [w1325 _] -> w39
    disable-tunnel: _ -> [w1324 _]
    frame Disabled {
      n1124 = while {
        tunnel: w1324 -> [_]
        tunnel: [w1326] -> w1325
        tunnel: [w1327] -> _
        i -> [w1327]
        stop <- w1326 stop-if-true
        w1343 = u16 10 items=["1.0"=10, "1.5"=15, "2.0"=20] ("stop bits (10: 1 bit)")
        n1125 = Wait (ms)(milliseconds to wait=u32 10) -> ()  [unwired: 1 out]
        n1126 = call-poly "VISA Configure Serial Port"("VISA resource name"=refnum<visa-resource-name> "ASRL1::INSTR" ("COM PORT"), "timeout (10sec)"=u32 10, "baud rate (9600)"=u32 57600, "data bits (8)"=u16 8, "stop bits (10: 1 bit)"=w1343) -> ("VISA resource name out"=w1329:refnum<visa-resource-name>, "error out"=w1338:errorcluster)  [unwired: 9 in]
        n1127 = VISA Read(VISA resource name=w1329, byte count=u32 2 ("byte count (0)")) -> (read buffer=w1337:string)  [unwired: 1 in, 3 out]
        n1128 = String Subset(string=w1337, offset (0)=0, length (rest)=2 ("length (rest)")) -> (substring=w1336:string)
        n1129 = Match Pattern(string=w1336, regular expression="<>") -> (offset past match=w1333:i32)  [unwired: 1 in, 3 out]
        n1130 = Greater Or Equal?(x=w1333, y=0) -> (x >= y?=w1328:bool)
        n1131 = case shown="True" w1328 {
          tunnel: w1329 -> [_ w1347]
          tunnel: w1338 -> [_ w1346]
          frame False {
          }
          frame True {
            n1132 = VISA Read(VISA resource name=w1347, byte count=u32 32 ("byte count (0)"), error in (no error)=w1346) -> (read buffer=w1345:string)  [unwired: 3 out]
            n1133 = String Subset(string=w1345, offset (0)=0, length (rest)=8 ("length (rest)")) -> (substring=w1349:string)
            n1134 = String Subset(string=w1345, offset (0)=8, length (rest)=8 ("length (rest)")) -> (substring=w1350:string)
            n1135 = Decimal String To Number(string=w1350) -> (number=w1357:i32)  [unwired: 2 in, 1 out]
            n1136 = Decimal String To Number(string=w1349) -> (number=w1353:i32)  [unwired: 2 in, 1 out]
            n1137 = Divide(x=w1357, y=10000) -> ()  [unwired: 1 out]
            n1138 = Divide(x=w1353, y=1000000) -> ()  [unwired: 1 out]
          }
        }
        n1139 = local read "Quit"() -> (w1326:bool)
      }
    }
    frame Enabled {
    }
  }
  n1140 = while {
    shift-right: [w1372] -> w52
    shift-left: _ -> [w1363]
    shift-right: [w1371] -> w51
    shift-left: errorcluster {"status"=TRUE, "code"=0, "source"="Init"} ("error IO") -> [w1365]
    tunnel: [w1360] -> w42
    tunnel: [w1370] -> _
    i -> [w1370]
    stop <- w1360 stop-if-true
    n1141 = local read "Com Port 1"() -> (w1364:refnum<visa-resource-name>)
    n1142 = Wait (ms)(milliseconds to wait=u32 10) -> ()  [unwired: 1 out]
    n1143 = local read "Port 1a"() -> (w1366:bool)
    n1144 = Unbundle(w1365) -> ("status"=→"Port 3":bool)  [unwired: 2 out]
    n1145 = local read "Port 3"() -> (w1367:bool)
    n1146 = Not Equal?(x=w1364, y=w1363) -> (x != y?=w1361:bool)
    n1147 = Or(x=w1367, y=w1366) -> (x .or. y?=w1369:bool)
    n1148 = case shown="True" w1361 {
      tunnel: [w1373 errorcluster {"status"=TRUE, "code"=0, "source"="Init"} ("error out")] -> w1362
      tunnel: w1365 -> [w1373 _]
      frame False {
      }
      frame True {
      }
    }
    n1149 = case shown="True" w1369 {
      frame False {
        w1375 = FALSE ("Visible")
        n1150 = property on="Port 1a" class="Bool (strict)"("Visible"=w1375) -> ()  [unwired: 2 in, 2 out]
        n1151 = property on="Port 3" class="Bool (strict)"("Visible"=w1375) -> ()  [unwired: 2 in, 2 out]
      }
      frame True {
        w1376 = TRUE ("Visible")
        n1152 = property on="Port 1a" class="Bool (strict)"("Visible"=w1376) -> ()  [unwired: 2 in, 2 out]
        n1153 = property on="Port 3" class="Bool (strict)"("Visible"=w1376) -> ()  [unwired: 2 in, 2 out]
      }
    }
    n1154 = case shown="No Error" w1362 {
      selector: w1362 -> [w1385 w1412]
      tunnel: [w1378 w1416] -> w1372
      tunnel: [w1387 w1410] -> w1371
      tunnel: w1363 -> [w1386 w1414]
      frame No Error {
        n1155 = property class="Instr"(reference=w1386, error in=w1385) -> (reference out=w1383:refnum<visa-resource-name>, error out=w1384:errorcluster, "Serial Settings:Number of Bytes at Serial Port"=w1379:u32)
        n1156 = while {
          tunnel: [w1405] -> w1387
          tunnel: [w1404] -> w1388
          tunnel: w1384 -> [w1403]
          tunnel: w1383 -> [w1402]
          stop <- TRUE stop-if-true
          n1157 = property class="Instr" props=["Serial Settings:Number of Bytes at Serial Port"](reference=w1402, error in=w1403) -> (reference out=w1407:refnum<visa-resource-name>, error out=w1406:errorcluster)  [unwired: 1 out]
          n1158 = VISA Read(VISA resource name=w1407, byte count=u32 1000, error in (no error)=w1406) -> (VISA resource name out=w1404:refnum<visa-resource-name>, read buffer=w1389:string, error out=w1405:errorcluster)  [unwired: 1 out]
          "UNI READ" <- w1389
          n1159 = Spreadsheet String To Array(delimiter (Tab)=";", format string="", spreadsheet string=w1389, array type (2D Dbl)=dbl[] []) -> (array=w1399:dbl[])
          n1160 = Index Array(array=w1399) -> (element #1=→"LVDT MIN":dbl, element #2=→"LVDT MAX":dbl, element #3=→"LVDT Peak":dbl, element #4=→"pizo raw":dbl, element #5=→"Friction":dbl, element #6=→"cof 2":dbl)  [unwired: 6 in]
        }
        n1161 = Greater?(x=w1379, y=u32 5) -> (0:w1381:bool)
        n1162 = Not(x=w1381) -> (.not. x?=→"Port 1a":bool)
        n1163 = VISA Flush I/O Buffer(VISA resource name=w1388) -> (VISA resource name out=w1378:refnum<visa-resource-name>, error out=→"error out 10":errorcluster)  [unwired: 2 in]
      }
      frame Error {
        w1422 = u16 0 items=["None", "XON/XOFF", "RTS/CTS", "XON/XOFF & RTS/CTS", "DTR/DSR", "XON/XOFF & DTR/DSR"] ("flow control (0:none)  2")
        w1420 = u16 10 items=["1.0"=10, "1.5"=15, "2.0"=20] ("stop bits 2")
        w1418 = u16 0 items=["None", "Odd", "Even", "Mark", "Space"] ("parity 2")
        w1419 = u32 10000  # timeout (10sec)
        n1164 = VISA Close(VISA resource name=w1414, error in (no error)=w1412) -> (error out=w1415:errorcluster)
        n1165 = local write "Port 1a"(FALSE ("Port 1a")) -> ()
        n1166 = call <vilib>:"Clear Errors.vi"("error in (no error)"=w1415) -> ("error out"=w1413:errorcluster)  [unwired: 5 in, 1 out]
        n1167 = local read "Com Port 1"() -> (w1409:refnum<visa-resource-name>)
        n1168 = call-poly "VISA Configure Serial Port"("VISA resource name"=w1409, "timeout (10sec)"=w1419, "baud rate (9600)"=u32 250000 ("baud rate  2"), "data bits (8)"=u16 8 ("data bits  2"), "parity (0:none)"=w1418, "error in (no error)"=w1413, "stop bits (10: 1 bit)"=w1420, "flow control (0:none)"=w1422) -> ("VISA resource name out"=w1423:refnum<visa-resource-name>, "error out"=w1424:errorcluster)  [unwired: 6 in]
        n1169 = flat-sequence {
          tunnel: w1423 -> [w1426]
          tunnel: w1424 -> [w1425]
          tunnel: [w1426] -> w1416
          tunnel: [w1425] -> w1410
          frame #0 {
            n1170 = Wait (ms)(milliseconds to wait=u32 50) -> ()  [unwired: 1 out]
          }
        }
        "Residual Uno" <- ""
        "Port 1 Error" <- w1410
      }
    }
    n1171 = local read "Quit"() -> (w1360:bool)
    "Error Uno" <- w1365
  }
  n1172 = while {
    stop <- w1433 stop-if-true
    # "V0OLTAGE TO STROKE (peice vise calibration)"
    n1173 = Wait (ms)(milliseconds to wait=u32 10) -> ()  [unwired: 1 out]
    n1174 = local read "LVDT Peak"() -> (w1430:dbl)
    n1175 = formula code="// Dynamic Parameterized Linear Interpolation Node\n// Inputs: vpp_val, voltages (Array), distances (Array)\n// Outputs: stroke\n\nint i = 0;\nint segments = 11; // 12 points make 11 interpolation segments\n\n// 1. Lower Boundary Clamp\nif (vpp_val <= voltages[0]) {\n    stroke = distances[0];\n}\n// 2. Upper Boundary Clamp\nelse if (vpp_val >= voltages[segments]) {\n    stroke = distances[segments];\n}\n// 3. Dynamic Segment Search Loop\nelse {\n    stroke = distances[0]; // Fallback baseline\n    for (i = 0; i < segments; i++) {\n        if (vpp_val >= voltages[i] && vpp_val <= voltages[i+1]) {\n            // Standard linear interpolation formula using array lookups\n            stroke = distances[i] + (vpp_val - voltages[i]) * (distances[i+1] - distances[i]) / (voltages[i+1] - voltages[i]);\n            break; // Segment found, safely exit the loop\n        }\n    }\n}"("vpp_val"=w1430, "voltages"="calibration values", "distances"="STROKE") -> ("stroke"=w1429:dbl)
    n1176 = local write "measured_stroke"(w1429) -> ()
    n1177 = local read "Quit"() -> (w1433:bool)
  }
  n1178 = while {
    stop <- w1453 stop-if-true
    # "SampleTemp;TagrgetSampleTemp;currentDutyCycle;AmbTemp;dacStatus;dacStatus;activeErrorCode;Kp;Ki;Kd;SampleRaw;AmbRaw"
    n1179 = call <vilib>:"High Resolution Polling Wait.vi"("seconds to wait"=0.02) -> ()  [unwired: 10 in, 1 out]
    n1180 = local read "Due read"() -> (w1451:string)
    n1181 = Spreadsheet String To Array(delimiter (Tab)=";", format string="", spreadsheet string=w1451, array type (2D Dbl)=string[] []) -> (array=w1435:string[])
    n1182 = Fract/Exp String To Number(string=w1435) -> (number=w1434:dbl[])  [unwired: 3 in, 1 out]
    n1183 = Index Array(array=w1434) -> (element #1=→"SampleTemp":dbl, element #2=→"TagrgetSampleTemp":dbl, element #3=→"currentDutyCycle":dbl, element #4=→"AmbTemp":dbl, element #5=→"dacStatus":dbl, element #6=→"VppStatus":dbl, element #7=→"activeErrorCode":dbl, element #8=→"Kp":dbl, element #9=→"Ki":dbl, element #10=→"Kd":dbl, element #11=→"SampleRaw":dbl, element #12=→"AmbRaw":dbl)  [unwired: 12 in]
    n1184 = local read "Quit"() -> (w1453:bool)
  }
  n1185 = while {
    shift-right: [w1467] -> w37
    shift-left: _ -> [w1458]
    shift-right: [w1466] -> w36
    shift-left: errorcluster {"status"=FALSE, "code"=0, "source"="Init"} ("error out") -> [w1460]
    tunnel: [w1455] -> w41
    tunnel: [w1465] -> _
    i -> [w1465]
    stop <- w1455 stop-if-true
    n1186 = local read "Com Port 2"() -> (w1459:refnum<visa-resource-name>)
    n1187 = local read "Port 2a"() -> (w1461:bool)
    n1188 = Unbundle(w1460) -> ("status"=→"Port 4":bool)  [unwired: 2 out]
    n1189 = call <vilib>:"High Resolution Polling Wait.vi"("seconds to wait"=0.02) -> ()  [unwired: 10 in, 1 out]
    n1190 = local read "Port 4"() -> (w1462:bool)
    n1191 = Not Equal?(x=w1459, y=w1458) -> (x != y?=w1457:bool)
    n1192 = Or(x=w1462, y=w1461) -> (x .or. y?=w1464:bool)
    n1193 = case shown="True" w1464 {
      frame False {
        w1470 = FALSE ("Visible")
        n1194 = property on="Port 2a" class="Bool (strict)"("Visible"=w1470) -> ()  [unwired: 2 in, 2 out]
        n1195 = property on="Port 4" class="Bool (strict)"("Visible"=w1470) -> ()  [unwired: 2 in, 2 out]
      }
      frame True {
        w1471 = TRUE ("Visible")
        n1196 = property on="Port 2a" class="Bool (strict)"("Visible"=w1471) -> ()  [unwired: 2 in, 2 out]
        n1197 = property on="Port 4" class="Bool (strict)"("Visible"=w1471) -> ()  [unwired: 2 in, 2 out]
      }
    }
    n1198 = case shown="True" w1457 {
      tunnel: [w1468 errorcluster {"status"=TRUE, "code"=0, "source"="Init"} ("error out")] -> w1456
      tunnel: w1460 -> [w1468 _]
      frame False {
      }
      frame True {
      }
    }
    n1199 = case shown="No Error" w1456 {
      selector: w1456 -> [w1482 w1513]
      tunnel: [w1475 w1518] -> w1467
      tunnel: [w1483 w1511] -> w1466
      tunnel: w1458 -> [w1485 w1516]
      frame No Error {
        n1200 = property class="Instr" props=["Serial Settings:Number of Bytes at Serial Port"](reference=w1485, error in=w1482) -> (reference out=w1476:refnum<visa-resource-name>, error out=w1481:errorcluster)  [unwired: 1 out]
        n1201 = while {
          tunnel: [w1493] -> w1477
          tunnel: [w1492] -> w1478
          tunnel: w1481 -> [w1491]
          tunnel: w1476 -> [w1490]
          tunnel: [w1489] -> _
          i -> [w1489]
          stop <- TRUE stop-if-true
          n1202 = property class="Instr" props=["Serial Settings:Number of Bytes at Serial Port"](reference=w1490, error in=w1491) -> (reference out=w1495:refnum<visa-resource-name>, error out=w1494:errorcluster)  [unwired: 1 out]
          n1203 = VISA Read(VISA resource name=w1495, byte count=u32 1000, error in (no error)=w1494) -> (VISA resource name out=w1492:refnum<visa-resource-name>, read buffer=→"Due read":string, error out=w1493:errorcluster)  [unwired: 1 out]
        }
        n1204 = local read "Command"() -> (w1473:string)
        n1205 = call <vilib>:"Trim Whitespace.vi"("string"=w1473) -> ("trimmed string"=w1472:string)  [unwired: 1 in]
        n1206 = Not Equal?(x=w1472, y="") -> (x != y?=w1479:bool)
        n1207 = case shown="True" w1479 {
          tunnel: w1478 -> [w1497 w1502]
          tunnel: [w1497 w1506] -> w1484
          tunnel: w1477 -> [w1496 w1501]
          tunnel: [w1496 w1504] -> w1483
          tunnel: w1472 -> [_ w1500]
          tunnel: [_ w1503] -> _
          frame False {
            # "DATA  WRITE LOOP"
          }
          frame True {
            n1208 = Concatenate Strings(w1500, "\r\n") -> (w1499:string)
            n1209 = VISA Write(VISA resource name=w1502, write buffer=w1499, error in (no error)=w1501) -> (VISA resource name out=w1506:refnum<visa-resource-name>, return count=w1503:u32, error out=w1505:errorcluster)
            n1210 = flat-sequence {
              tunnel: w1505 -> [w1508]
              tunnel: [w1508] -> w1504
              frame #0 {
                n1211 = local write "Command"("" ("Command")) -> ()
                n1212 = Wait (ms)(milliseconds to wait=u32 5) -> ()  [unwired: 1 out]
              }
            }
          }
        }
        n1213 = VISA Flush I/O Buffer(VISA resource name=w1484) -> (VISA resource name out=w1475:refnum<visa-resource-name>, error out=→"error out 9":errorcluster)  [unwired: 2 in]
      }
      frame Error {
        w1524 = u16 0 items=["None", "XON/XOFF", "RTS/CTS", "XON/XOFF & RTS/CTS", "DTR/DSR", "XON/XOFF & DTR/DSR"] ("flow control (0:none)  2")
        w1522 = u16 10 items=["1.0"=10, "1.5"=15, "2.0"=20] ("stop bits 2")
        w1520 = u16 0 items=["None", "Odd", "Even", "Mark", "Space"] ("parity 2")
        w1521 = u32 10000  # timeout (10sec)
        n1214 = VISA Clear(VISA resource name=w1516, error in (no error)=w1513) -> (VISA resource name out=w1515:refnum<visa-resource-name>, error out=w1514:errorcluster)
        n1215 = VISA Close(VISA resource name=w1515, error in (no error)=w1514) -> (error out=w1517:errorcluster)
        n1216 = call <vilib>:"Clear Errors.vi"("error in (no error)"=w1517) -> ()  [unwired: 5 in, 2 out]
        n1217 = local read "Com Port 2"() -> (w1510:refnum<visa-resource-name>)
        "visa due" <- w1510
        n1218 = call-poly "VISA Configure Serial Port"("VISA resource name"=w1510, "timeout (10sec)"=w1521, "baud rate (9600)"=u32 250000 ("baud rate  2"), "data bits (8)"=u16 8 ("data bits  2"), "parity (0:none)"=w1520, "stop bits (10: 1 bit)"=w1522, "flow control (0:none)"=w1524) -> ("VISA resource name out"=w1525:refnum<visa-resource-name>, "error out"=w1526:errorcluster)  [unwired: 7 in]
        n1219 = flat-sequence {
          tunnel: w1525 -> [w1528]
          tunnel: w1526 -> [w1527]
          tunnel: [w1528] -> w1518
          tunnel: [w1527] -> w1511
          frame #0 {
            n1220 = Wait (ms)(milliseconds to wait=u32 50) -> ()  [unwired: 1 out]
          }
        }
        "Residual Due" <- ""
        "Port 2 Error" <- w1511
      }
    }
    n1221 = local read "Quit"() -> (w1455:bool)
    "Error Due" <- w1460
  }
  n1222 = local write "FRICVALZ"(0.0 ("FRICVALZ")) -> ()
  n1223 = property on="RUN" class="Bool (strict)"("Visible"=TRUE) -> ()  [unwired: 2 in, 2 out]
  n1224 = while {
    tunnel: [w1545] -> _
    tunnel: [w1530] -> w54
    i -> [w1545]
    stop <- w1530 stop-if-true
    n1225 = local read "conststatus"() -> (w1534:dbl)
    n1226 = local read "Main Tab"() -> (w1532:T2)
    n1227 = local read "EDIT"() -> (w1551:bool)
    n1228 = local read "Rate"() -> (w1550:dbl)
    n1229 = case shown="True" w1551 {
      tunnel: [FALSE TRUE] -> w1537
      frame False {
      }
      frame True {
      }
    }
    n1230 = property on="Time slide" class="Slide (strict)"("Scale.Range:Maximum"=2500.0) -> ()  [unwired: 2 in, 2 out]
    n1231 = Equal?(x=w1532, y=T23."About" ("Main Tab")) -> (x = y?=w1543:bool)
    n1232 = Equal?(x=w1534, y=0.0) -> (x = y?=w1535:bool)
    n1233 = Divide(x=1.0, y=w1550) -> (x/y=w1546:dbl)
    "Time 2" <- w1546
    n1234 = case shown="True" w1535 {
      frame False {
      }
      frame True {
        # "C:\\WinDucom\\calibrate WO 2391.dcf"
        n1235 = local write "Lan flag"(22) -> ()
        n1236 = local write "conststatus"(10.0 ("rpm value : 2")) -> ()
        n1237 = String To Path(string="C:\\LAB-IQ\\calibrate WO 2465.dcf") -> (path=w1557:path)
        n1238 = Open/Create/Replace File "Open File"(file path (use dialog)=w1557) -> (refnum out=w1555:refnum<file>)  [unwired: 5 in, 2 out]
        n1239 = for {
          N: 23 -> [_]
          tunnel: w1555 -> [w1566]
          i -> [w1560]
          (unwired) TRUE ("line mode (F)")
          n1240 = Read from Text File "Read File"(file (use dialog)=w1566) -> (text=w1565:string)  [unwired: 3 in, 3 out]
          n1241 = Match Pattern(string=w1565, regular expression="]") -> (after substring=w1563:string)  [unwired: 1 in, 3 out]
          n1242 = String Subset(string=w1565, offset (0)=5, length (rest)=10 ("length (rest)")) -> (substring=w1558:string)
          n1243 = Fract/Exp String To Number(string=w1558) -> (number=w1559:dbl)  [unwired: 3 in, 1 out]
          n1244 = Match Pattern(string=w1563, regular expression="-") -> (before substring=w1561:string)  [unwired: 1 in, 3 out]
          n1245 = case shown="5" w1560 {
            tunnel: w1559 -> [w1569 w1570 w1571 w1572 _ _ _ w1577 w1578 _ w1579 w1580 w1581 w1582 w1583 w1584 _ w1585 w1586 _ _ _ _ _]
            tunnel: w1561 -> [_ _ _ _ w1573 w1574 w1575 _ _ _ _ _ _ _ _ _ _ _ _ w1587 w1588 _ w1589 _]
            frame 0 {
              n1246 = local write "FRIC. FORCE :"(w1569) -> ()
            }
            frame 1 {
              n1247 = local write "TEMPERATURE :"(w1570) -> ()
            }
            frame 2 {
              n1248 = local write "HUMIDITY:"(w1571) -> ()
            }
            frame 3 {
              n1249 = local write "AIR TEMPERATURE :"(w1572) -> ()
            }
            frame 4 {
              n1250 = local write "Com Port 1"(w1573) -> ()
            }
            frame 5 {
              n1251 = local write "Com Port 2"(w1574) -> ()
              n1252 = local write "visa due"(w1574) -> ()
            }
            frame 6 {
              n1253 = String To Path(string=w1575) -> (path=w1576:path)
              n1254 = local write "File Path"(w1576) -> ()
              "String" <- w1575
            }
            frame 7 {
              n1255 = local write "DISPLACEMENT :"(w1577) -> ()
            }
            frame 8 {
              n1256 = local write "STROKE GAIN :"(w1578) -> ()
            }
            frame 9 {
            }
            frame 10 {
              n1257 = local write "Language Selection"(w1579) -> ()
            }
            frame 11 {
              n1258 = local write "CH-POWER +"(w1580) -> ()
            }
            frame 12 {
              n1259 = local write "CH-POWER -"(w1581) -> ()
            }
            frame 13 {
              n1260 = local write "CH-HEATER"(w1582) -> ()
            }
            frame 14 {
              n1261 = local write "CH-HUMIDITY WET"(w1583) -> ()
            }
            frame 15 {
              n1262 = local write "CH-HUMIDITY DRY"(w1584) -> ()
            }
            frame 16 {
            }
            frame 17 {
              n1263 = local write "AIR TEMP INTERCEPT:"(w1585) -> ()
            }
            frame 18 {
              n1264 = local write "TEMP INTERCEPT:"(w1586) -> ()
            }
            frame 19 {
              n1265 = local write "S.NO"(w1587) -> ()
            }
            frame 20 {
              n1266 = local write "Com Port 3"(w1588) -> ()
            }
            frame 21 {
            }
            frame 22 {
              n1267 = local write "C3 :"(w1589) -> ()
            }
            frame 23, Default {
            }
          }
        }
      }
    }
    n1268 = Select(t=u32 2500 ("milliseconds to wait"), s=w1543, f=u32 500 ("milliseconds to wait")) -> (s? t:f=w1541:u32)
    n1269 = Multiply(x=w1546, y=w1541) -> (x*y=w1548:dbl)
    n1270 = property on="Time slide" class="Slide (strict)"("Visible"=w1537) -> ()  [unwired: 2 in, 2 out]
    n1271 = call "Elapsed Time2"("Time Target (s)"=w1548, "Auto Reset"=TRUE) -> ("Time has Elapsed"=w1538:bool)  [unwired: 10 in, 7 out]
    n1272 = case shown="True" w1538 {
      frame False {
      }
      frame True {
        n1273 = stacked-sequence {
          frame #0 {
            # "DATA PROCESSING"
            # "115 mV/N"
            n1274 = local read "AmbTemp"() -> (→"AIR TEMP":dbl)
            n1275 = local read "SampleTemp"() -> (w1592:dbl)
            "TEMP 2" <- w1592
            "TEMP 3" <- w1592
            n1276 = local read "RH Numeric:"() -> (w1598:dbl)
            n1277 = local read "HUMIDITY:"() -> (w1599:dbl)
            n1278 = local read "FRICVALZ"() -> (w1609:dbl)
            n1279 = local read "Friction"() -> (w1594:dbl)
            n1280 = local write "TEMP"(w1592) -> ()
            n1281 = Multiply(x=w1598, y=w1599) -> (x*y=→"Humidity ( %RH )" →"Hum" →"Hum 2":dbl)
            n1282 = Subtract(x=w1594, y=w1609) -> (x-y=w1604:dbl)
            "FF 2" <- w1604
            "FF 4" <- w1604
